vi "Scan CSM-VI.vi"(6 "Config Path":path, 7 "Block Diagram Window:Window Bounds":T1, 8 "Error In":errorcluster caption="Error in (no error)", 11 "Root":path) -> (0 "Error Out":errorcluster)   [LabVIEW 2017]
uses:
  <vilib>/Utility/miscctls.llb/LVRectTypeDef.ctl
  _csmHelper/API with lvcsm Support/CSM-Helper API with lvcsm Support.lvlib
  _ui/csm-ui-support.lvlib
panel:
  in  "Termiate":bool
  out "Path":path
  out "Slide":i32(slide) scale=0.0..2506.0
  out "All Files in Dir":path[](array[path])
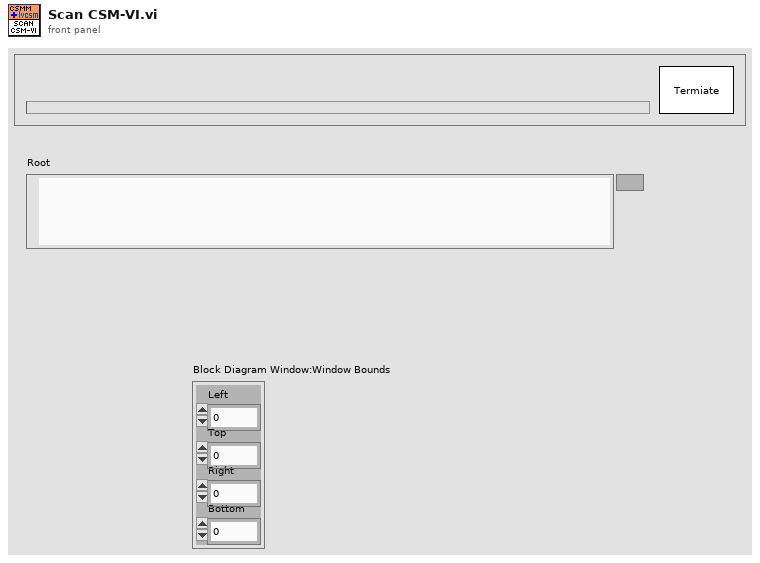
[diagram p1: front panel]
types:
  T1 = typedef "LVRectTypeDef.ctl" = cluster{"Left":i16, "Top":i16, "Right":i16, "Bottom":i16}
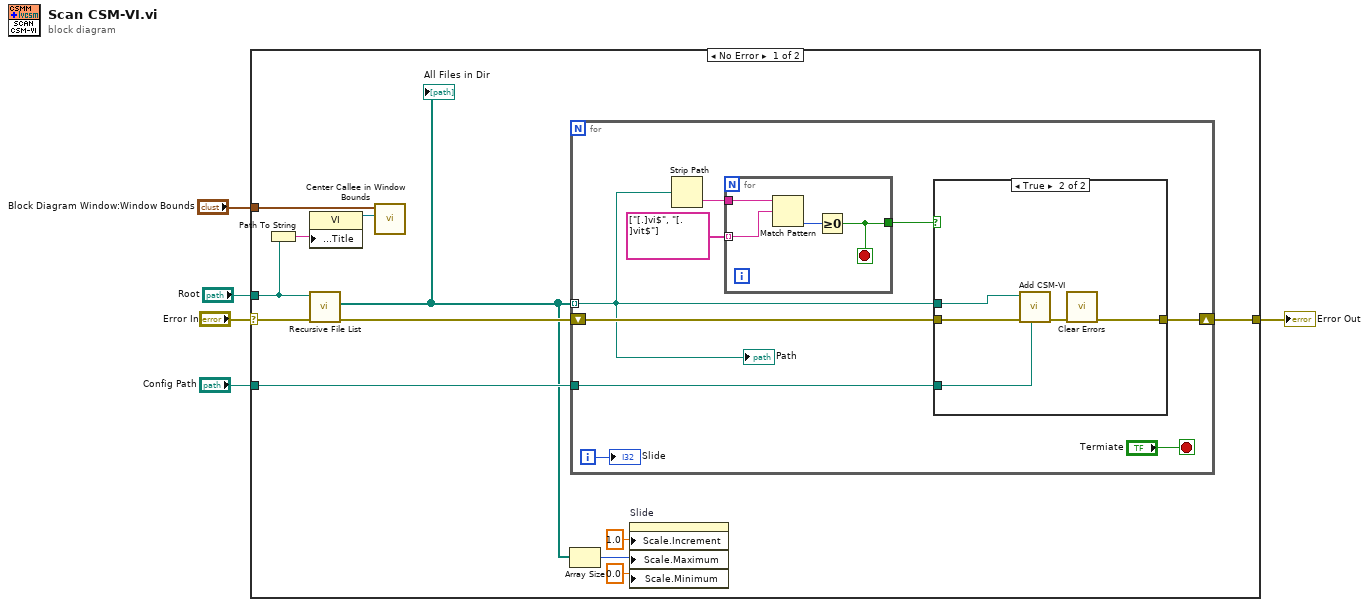
[diagram p0: block diagram]
diagram:
  n1 = case shown="No Error" "Error In" {
    selector: "Error In" -> [w17 w37]
    tunnel: [w14 w37] -> w4
    tunnel: "Config Path" -> [w16 _]
    tunnel: "Root" -> [w11 _]
    tunnel: "Block Diagram Window:Window Bounds" -> [w6 _]
    frame No Error {
      n2 = Path To String(path=w11) -> (string=w12:string)
      n3 = property class="VI"("Front Panel.Title"=w12) -> (reference out=w7:refnum<vi>)  [unwired: 2 in, 1 out]
      n4 = call <vilib>:"Recursive File List.vi"("error in (no error)"=w17, "Folder Path"=w11) -> ("error out"=w15:errorcluster, "All Files in Dir"=w13:path[])  [unwired: 5 in, 3 out]
      "All Files in Dir" <- w13
      n5 = call "Center Callee in Window Bounds.vi"("Callee VI Refnum (Caller)"=w7, "Block Diagram Window:Window Bounds"=w6) -> ()  [unwired: 9 in, 1 out]
      n6 = Array Size(array=w13) -> (size(s)=w10:i32)
      n7 = for {
        tunnel: w13 -> [w20] mode=indexing
        tunnel: w16 -> [w26]
        shift-right: [w21] -> w14
        shift-left: w15 -> [w22]
        i -> [w19]
        stop <- "Termiate" stop-if-true
        n8 = Strip Path(path=w20) -> (name=w25:string)  [unwired: 1 out]
        n9 = for {
          tunnel: w25 -> [w36]
          tunnel: string[] ["[.]vi$", "[.]vit$"] ("name") -> [w35] mode=indexing
          tunnel: [w33] -> w23
          stop <- w33 stop-if-true
          n10 = Match Pattern(string=w36, regular expression=w35) -> (offset past match=w34:i32)  [unwired: 1 in, 3 out]
          n11 = Greater Or Equal To 0?(x=w34) -> (x >= 0?=w33:bool)
        }
        n12 = case shown="True" w23 {
          tunnel: w26 -> [_ w32]
          tunnel: w20 -> [_ w31]
          tunnel: w22 -> [w27 w30]
          tunnel: [w27 w28] -> w21
          frame False {
          }
          frame True {
            n13 = call "Add CSM-VI.vi"("Config Path"=w32, "error in (no error)"=w30, "CSM-VI"=w31) -> ("error out"=w29:errorcluster)  [unwired: 8 in]
            n14 = call <vilib>:"Clear Errors.vi"("error in (no error)"=w29) -> ("error out"=w28:errorcluster)  [unwired: 5 in, 1 out]
          }
        }
        "Path" <- w20
        "Slide" <- w19
      }
      n15 = property on="Slide" class="Slide (strict)"("Scale.Increment"=1.0 ("Scale.Range:Increment"), "Scale.Maximum"=w10, "Scale.Minimum"=0.0 ("Scale.Range:Minimum")) -> ()  [unwired: 2 in, 2 out]
    }
    frame Error {
    }
  }
  "Error Out" <- w4
